vi "4K_Probe_Pt_Dir_Amy_Jan2018_withdT.vi"() -> ()   [LabVIEW 2013]
uses:
  <vilib>/Utility/file.llb/Read From Spreadsheet File (DBL).vi
panel:
  out "T graph":cluster{"Y":dbl[], "Y":dbl[]}[](graph)
  out "Raw Samp Y":dbl
  out "Loci-in Samp Y":dbl
  out "LED":bool=TRUE caption="Enable"
  out "Y Comonent":cluster{"Y":dbl[], "Y":dbl[]}[](graph)
  out "Resis in KO":dbl
  in  "Thermometer Current":dbl
  out "Lock-in Temp":dbl
  in  "Write Data":bool=TRUE caption="Enable"
  in  "temp ratio":dbl
  out "Lock-in Samp X":dbl
  out "Raw Temp":dbl
  out "Raw Samp X":dbl
  out "X Component":cluster{"Y":dbl[], "Y":dbl[]}[](graph)
  in  "samp ratio":dbl
  in  "sampling rate":dbl=100.0
  in  "buffer":i32=1000
  in  "stop":bool
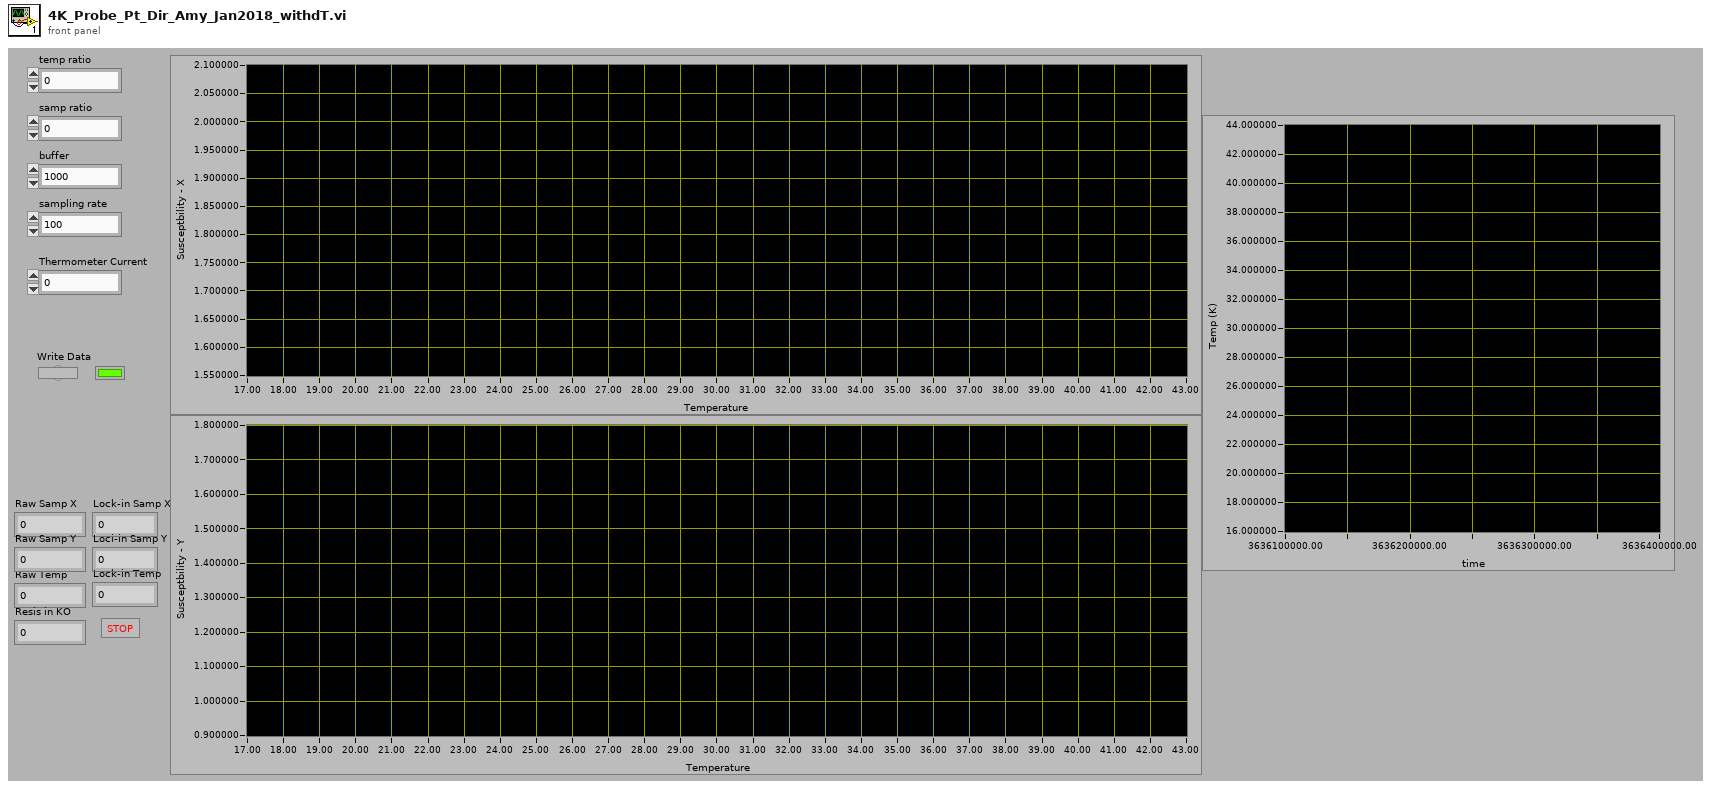
[diagram p1: front panel]
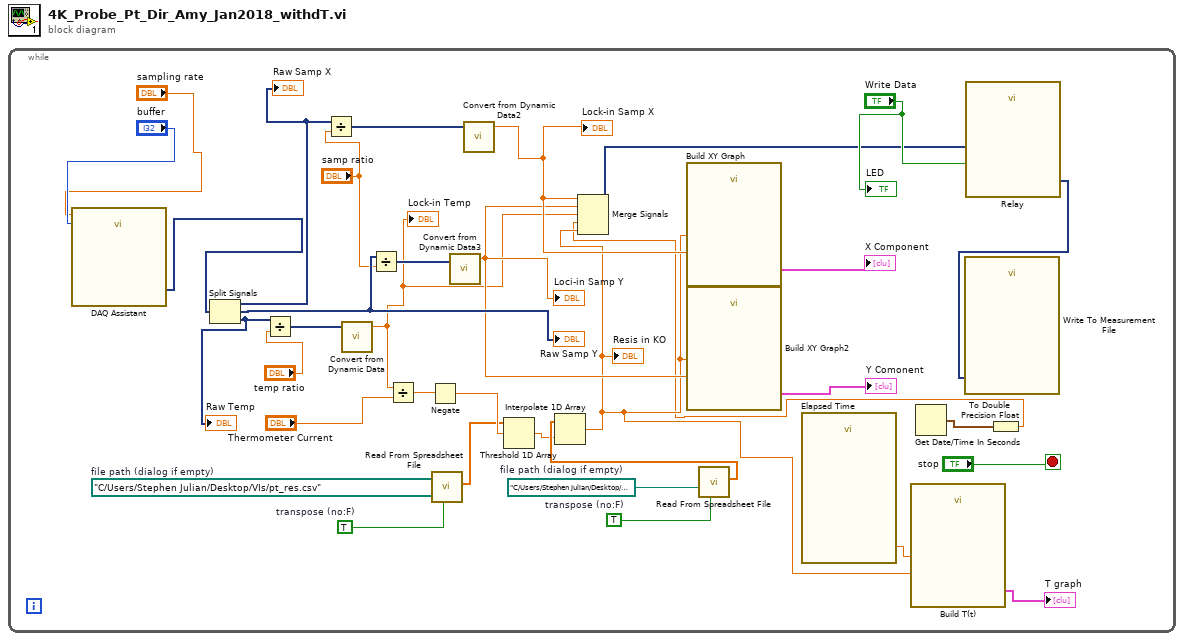
[diagram p0: block diagram]
diagram:
  n1 = while {
    stop <- "stop" stop-if-true
    w15 = TRUE  # transpose (no:F)
    w16 = path "C:/Users/Stephen Julian/Desktop/VIs/pt_temp.csv"  # file path (dialog if empty)
    w17 = TRUE  # transpose (no:F)
    w18 = path "C:/Users/Stephen Julian/Desktop/VIs/pt_res.csv"  # file path (dialog if empty)
    n2 = call "DAQ Assistant"("rate"="sampling rate", "number of samples"="buffer") -> ("data"=w10:dynamicdata)  [unwired: 15 in, 2 out]
    n3 = Split Signals(w10) -> (w34:dynamicdata, w28:dynamicdata, w29:dynamicdata)  [unwired: 3 out]
    "Raw Samp X" <- w34
    "Raw Temp" <- w29
    "Raw Samp Y" <- w28
    n4 = Divide(x=w29, y="temp ratio") -> (x/y=w19:dynamicdata)
    n5 = Divide(x=w34, y="samp ratio") -> (x/y=w21:dynamicdata)
    n6 = call "Convert from Dynamic Data"("Dynamic Data Type"=w19) -> ("Scalar"=w5:dbl)  [unwired: 1 in, 2 out]
    "Lock-in Temp" <- w5
    n7 = Divide(x=w28, y="samp ratio") -> (x/y=w20:dynamicdata)
    n8 = Divide(x=w5, y="Thermometer Current") -> (x/y=w12:dbl)
    n9 = Negate(x=w12) -> (-x=w11:dbl)
    n10 = call-poly <vilib>:"Read From Spreadsheet File.vi"("transpose (no:F)"=w17, "file path (dialog if empty)"=w18) -> ("first row"=w7:dbl[])  [unwired: 2 in, 7 out]
    n11 = call "Convert from Dynamic Data3"("Dynamic Data Type"=w20) -> ("Scalar"=w24:dbl)  [unwired: 1 in, 2 out]
    "Loci-in Samp Y" <- w24
    n12 = call "Convert from Dynamic Data2"("Dynamic Data Type"=w21) -> ("Scalar"=w30:dbl)  [unwired: 1 in, 2 out]
    "Lock-in Samp X" <- w30
    n13 = Threshold 1D Array(2:w11, 3:w7) -> (0:w13:dbl)  [unwired: 1 out]
    n14 = call-poly <vilib>:"Read From Spreadsheet File.vi"("transpose (no:F)"=w15, "file path (dialog if empty)"=w16) -> ("first row"=w14:dbl[])  [unwired: 2 in, 7 out]
    n15 = Interpolate 1D Array(1:w13, 2:w14) -> (0:w4:dbl)
    "Resis in KO" <- w4
    n16 = call "Build XY Graph"("Y Input"=w30, "X Input"=w4) -> ("XY Graph"=→"X Component":cluster{"Y":dbl[], "Y":dbl[]}[])  [unwired: 3 in, 6 out]
    n17 = call "Build XY Graph2"("Y Input"=w24, "X Input"=w4) -> ("XY Graph"=→"Y Comonent":cluster{"Y":dbl[], "Y":dbl[]}[])  [unwired: 3 in, 6 out]
    n18 = call "Elapsed Time"() -> ("Present (s)"=w3:dbl)  [unwired: 12 in, 7 out]
    n19 = call "Build T(t)"("Y Input"=w4, "X Input"=w3) -> ("XY Graph"=→"T graph":cluster{"Y":dbl[], "Y":dbl[]}[])  [unwired: 3 in, 6 out]
    n20 = Get Date/Time In Seconds() -> (seconds since 1Jan1904=w2:timestamp)
    n21 = To Double Precision Float(number=w2) -> (double precision float=w1:dbl)
    n22 = Merge Signals(w30, w24, w5, w1, w4) -> (w32:dynamicdata)
    n23 = call "Relay"("Enable"="Write Data", "Signals"=w32) -> ("Result"=w31:dynamicdata)  [unwired: 1 in, 8 out]
    n24 = call "Write To Measurement File"("Signals"=w31) -> ()  [unwired: 6 in, 13 out]
    "LED" <- "Write Data"
  }
